vi "DockerTools - Stop container by ID.vi"(8 "error in":errorcluster, 11 "Container ID":string) -> (0 "error out":errorcluster)   [LabVIEW 2017]
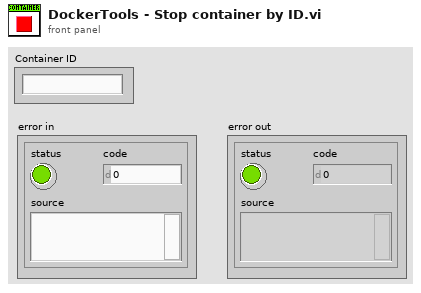
[diagram p1: front panel]
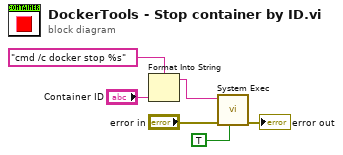
[diagram p0: block diagram]
diagram:
  n1 = Format Into String(format string="cmd /c docker stop %s" ("command line"), "Container ID") -> (resulting string=w2:string)  [unwired: 2 in, 1 out]
  n2 = call <vilib>:"System Exec.vi"("run minimized? (F)"=TRUE, "error in (no error)"="error in", "command line"=w2) -> ("error out"=→"error out":errorcluster)  [unwired: 5 in, 3 out]
